vi "Get COM by Descriptor.vi"(8 "error in (no error)":errorcluster, 10 "Generate error if no COM port found? (False)":bool, 11 "COM descriptor":string) -> (0 "error out":errorcluster, 1 "First COM port":T1, 2 "COM ports count":i32, 3 "COM list":T1[](array[typedef]))   [LabVIEW 2020, in "Get COM Descriptor.lvlib"]
doc: "Get list of COM ports matching given descriptor."
uses:
  Get COM Descriptor.lvlib
  COM port.ctl
  <vilib>/Utility/error.llb/Error Cluster From Error Code.vi
  <vilib>/ErrorRing/Error Ring.xnode
  get_com_descriptor.dll
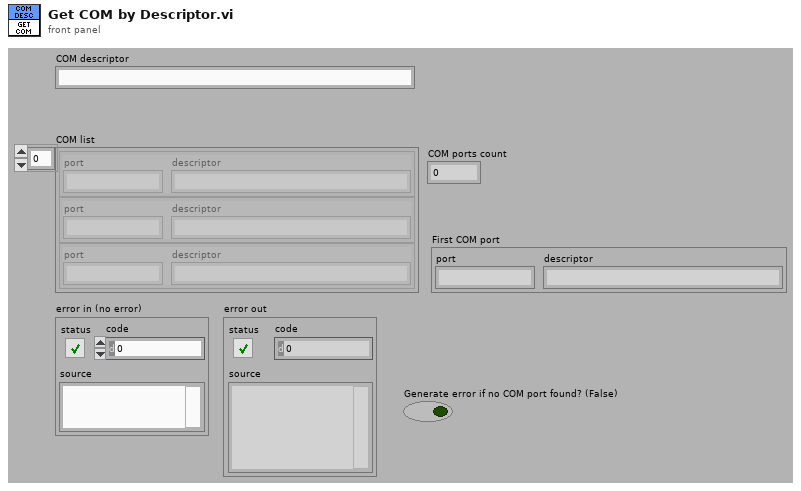
[diagram p1: front panel]
types:
  T1 = typedef "Get COM Descriptor.lvlib/COM port.ctl" = cluster{"port":string, "descriptor":string}
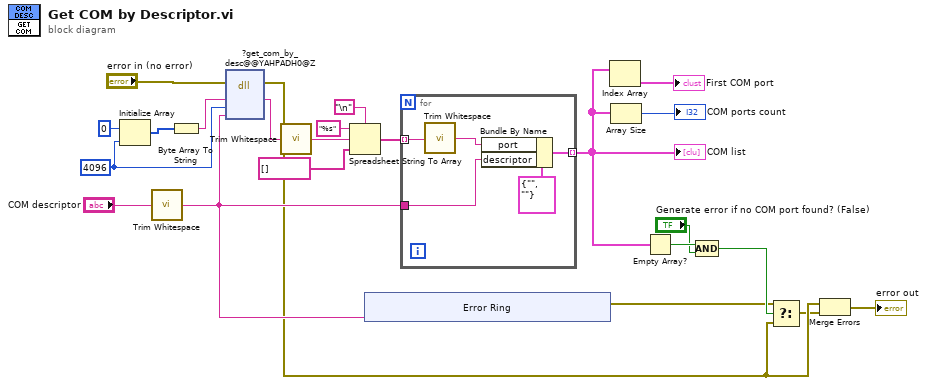
[diagram p0: block diagram]
diagram:
  w19 = 4096 ("dimension size")
  n1 = Initialize Array(u8 0 ("element"), w19) -> (w22:u8[])
  n2 = call <vilib>:"Trim Whitespace.vi"("string"="COM descriptor") -> ("trimmed string"=w9:string)  [unwired: 1 in]
  n3 = Byte Array To String(unsigned byte array=w22) -> (string=w20:string)
  n4 = dll-call lib="F:/z-bridge-v4/other/get_com_descriptor/get_com_descriptor.dll" fn="?get_com_by_desc@@YAHPADH0@Z"(error in="error in (no error)", "buf"=w20, "size"=w19, "desc"=w9) -> (error out=w3:errorcluster, "buf"=w18:string)  [unwired: 5 in, 1 out]
  n5 = call <vilib>:"Trim Whitespace.vi"("string"=w18) -> ("trimmed string"=w17:string)  [unwired: 1 in]
  n6 = Spreadsheet String To Array(delimiter (Tab)="\n", format string="%s", spreadsheet string=w17, array type (2D Dbl)=string[] []) -> (array=w14:string[])
  n7 = xnode "Error Ring"("parameter 0"=w9) -> ("error out"=w4:errorcluster)
  n8 = for {
    tunnel: w14 -> [w28] mode=indexing
    tunnel: [w26] -> w8 mode=indexing
    tunnel: w9 -> [w24]
    n9 = call <vilib>:"Trim Whitespace.vi"("string"=w28) -> ("trimmed string"=w25:string)  [unwired: 1 in]
    n10 = Bundle By Name(cluster=T1 {"port"="", "descriptor"=""} ("COM port"), "port"=w25, "descriptor"=w24) -> (w26:T1)
  }
  "COM list" <- w8
  n11 = Index Array(array=w8) -> (element=→"First COM port":T1)  [unwired: 1 in]
  n12 = Array Size(array=w8) -> (size(s)=→"COM ports count":i32)
  n13 = Empty Array?(array=w8) -> (empty?=w7:bool)
  n14 = Compound Arithmetic op=AND(w7, "Generate error if no COM port found? (False)") -> (w5:bool)
  n15 = Select(t=w4, s=w5, f=w3) -> (s? t:f=w2:errorcluster)
  n16 = Merge Errors(w3, w2) -> (→"error out":errorcluster)
